vi "ProximalSpeedAdjust.vi"(0 "MDF X Position":dbl, 1 "MDF Y Position":dbl, 2 "GPS X Position":dbl, 3 "GPS Y Position":dbl, 4 "MDF Speed":i32) -> (5 "Desired Speed Out":i32)   [LabVIEW 2014]
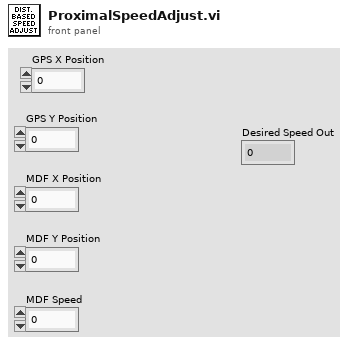
[diagram p1: front panel]
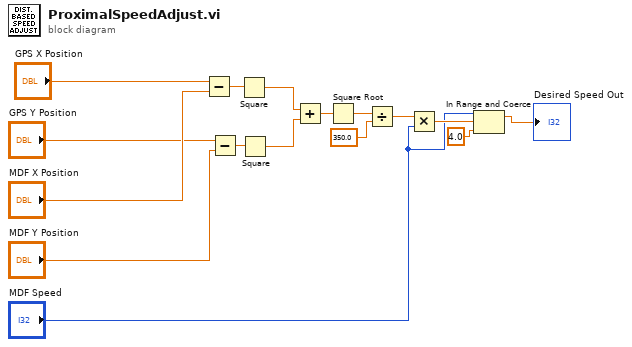
[diagram p0: block diagram]
diagram:
  n1 = Subtract(x="GPS X Position", y="MDF X Position") -> (x-y=w12:dbl)
  n2 = Subtract(x="GPS Y Position", y="MDF Y Position") -> (x-y=w11:dbl)
  n3 = Square(x=w12) -> (x^2=w10:dbl)
  n4 = Square(x=w11) -> (x^2=w9:dbl)
  n5 = Add(x=w10, y=w9) -> (x+y=w8:dbl)
  n6 = Square Root(x=w8) -> (sqrt(x)=w6:dbl)
  n7 = Divide(x=w6, y=350.0) -> (x/y=w5:dbl)
  n8 = Multiply(x=w5, y="MDF Speed") -> (x*y=w4:dbl)
  n9 = In Range and Coerce(upper limit="MDF Speed", x=w4, lower limit=4.0) -> (coerced(x)=→"Desired Speed Out":dbl)  [unwired: 1 out]
